vi "ExampleCalls.vi"() -> ()   [LabVIEW 2017]
uses:
  b0020f75-1b8a-49d1-8113-c99f900d1d2c.vi
  4e506ff5-569d-4df4-88c4-736d69b0cfc9.vi
  92922405-4113-4384-856e-a78ee2898198.vi
  Malleable VIs Basics Lesson 1.vi
panel:
  out "millisecond timer value":u32
  out "error out":errorcluster
  in  "error in (no error)":errorcluster
  out "notification 2":string
  out "notification":bool
  # "Open the block diagram!"
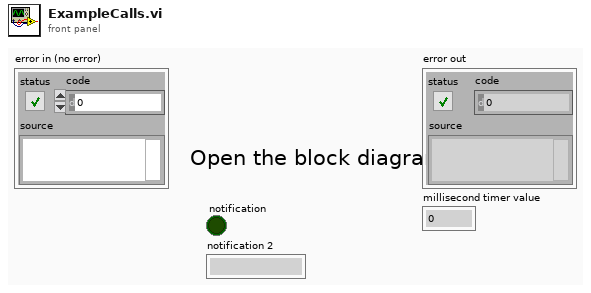
[diagram p1: front panel]
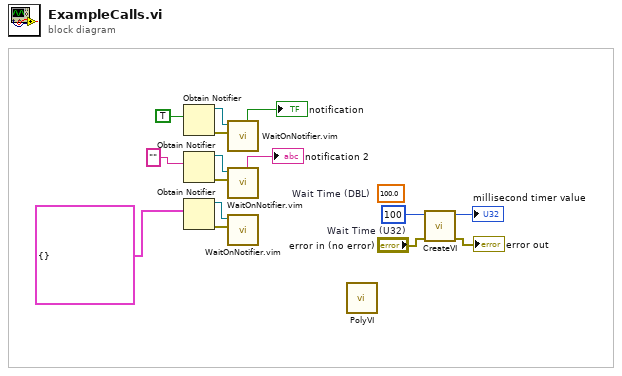
[diagram p0: block diagram]
diagram:
  (unwired) 100.0  # Wait Time (DBL)
  w1 = u32 100  # Wait Time (U32)
  n1 = Obtain Notifier(notification data type=TRUE) -> (notifier out=w13:refnum<notifier>, error out=w12:errorcluster)  [unwired: 3 in, 1 out]
  n2 = Obtain Notifier(notification data type="") -> (notifier out=w14:refnum<notifier>, error out=w11:errorcluster)  [unwired: 3 in, 1 out]
  n3 = Obtain Notifier(notification data type=cluster{} {}) -> (notifier out=w15:refnum<notifier>, error out=w10:errorcluster)  [unwired: 3 in, 1 out]
  n4 = call "WaitOnNotifier.vim"("error in (no error)"=w12, "notifier"=w13) -> ("notification"=→"notification":bool)  [unwired: 7 in, 2 out]
  n5 = call "WaitOnNotifier.vim"("error in (no error)"=w11, "notifier"=w14) -> ("notification"=→"notification 2":string)  [unwired: 7 in, 2 out]
  n6 = call "WaitOnNotifier.vim"("error in (no error)"=w10, "notifier"=w15) -> ()  [unwired: 7 in, 3 out]
  n7 = call-poly "PolyVI.vi"() -> ()  [unwired: 11 in, 1 out]
  n8 = call "CreateVI.vi"("error in (no error)"="error in (no error)", "Wait Time (ms)"=w1) -> ("error out"=→"error out":errorcluster, "millisecond timer value"=→"millisecond timer value":u32)  [unwired: 8 in]
